vi "server.Get Response Tree.vi"(8 "error in (no error)":errorcluster, 11 "JSONRPC Server in":refnum<class "JSONRPC Server.lvclass">) -> (0 "error out":errorcluster, 2 "Response Queue":refnum<data-value>, 3 "JSONRPC Server out":refnum<class "JSONRPC Server.lvclass">)   [LabVIEW 2016, in "JSONRPC Server.lvclass"]
uses:
  JSONRPC Server.lvclass
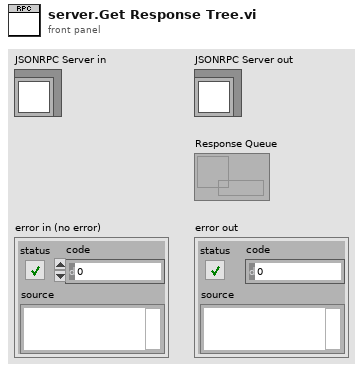
[diagram p1: front panel]
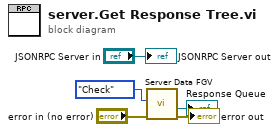
[diagram p0: block diagram]
diagram:
  n1 = call "Server Data FGV.vi"("error in (no error)"="error in (no error)", "Action"=enum16{"Initialize", "Check", "Close"}."Check") -> ("error out"=→"error out":errorcluster, "Responses Ref"=→"Response Queue":refnum<data-value>)  [unwired: 6 in, 2 out]
  "JSONRPC Server out" <- "JSONRPC Server in"
